vi "Preprocessing.vi"() -> (0 "Timestamp":dbl[](array[numeric]), 1 "Potência instantänea A":dbl[](array[numeric]), 2 "Potência Ativa B":dbl[](graph), 3 "Potência Ativa C":dbl[](graph))   [LabVIEW 2020]
uses:
  <vilib>/numeric/Random Number (Range) U64.vi
  <vilib>/numeric/Random Number (Range) DBL.vi
  <vilib>/numeric/sub_Random U32.vi
panel:
  out "Fator de potência":dbl
  in  "Limite inferior FP":dbl
  in  "Limite superior FP":dbl=100.0
  out "Corrente A":dynamicdata(graph)
  out "Tensão  C":dynamicdata(graph)
  out "Corrente C":dynamicdata(graph)
  out "Tensão B":dynamicdata(graph)
  out "Corrente B":dynamicdata(graph)
  out "Potência Ativa A":dbl[](graph)
  out "Corrente A":dbl[](array[numeric])
  out "Tensão A":dynamicdata(graph)
  out "Tensão A":dbl[](array[numeric])
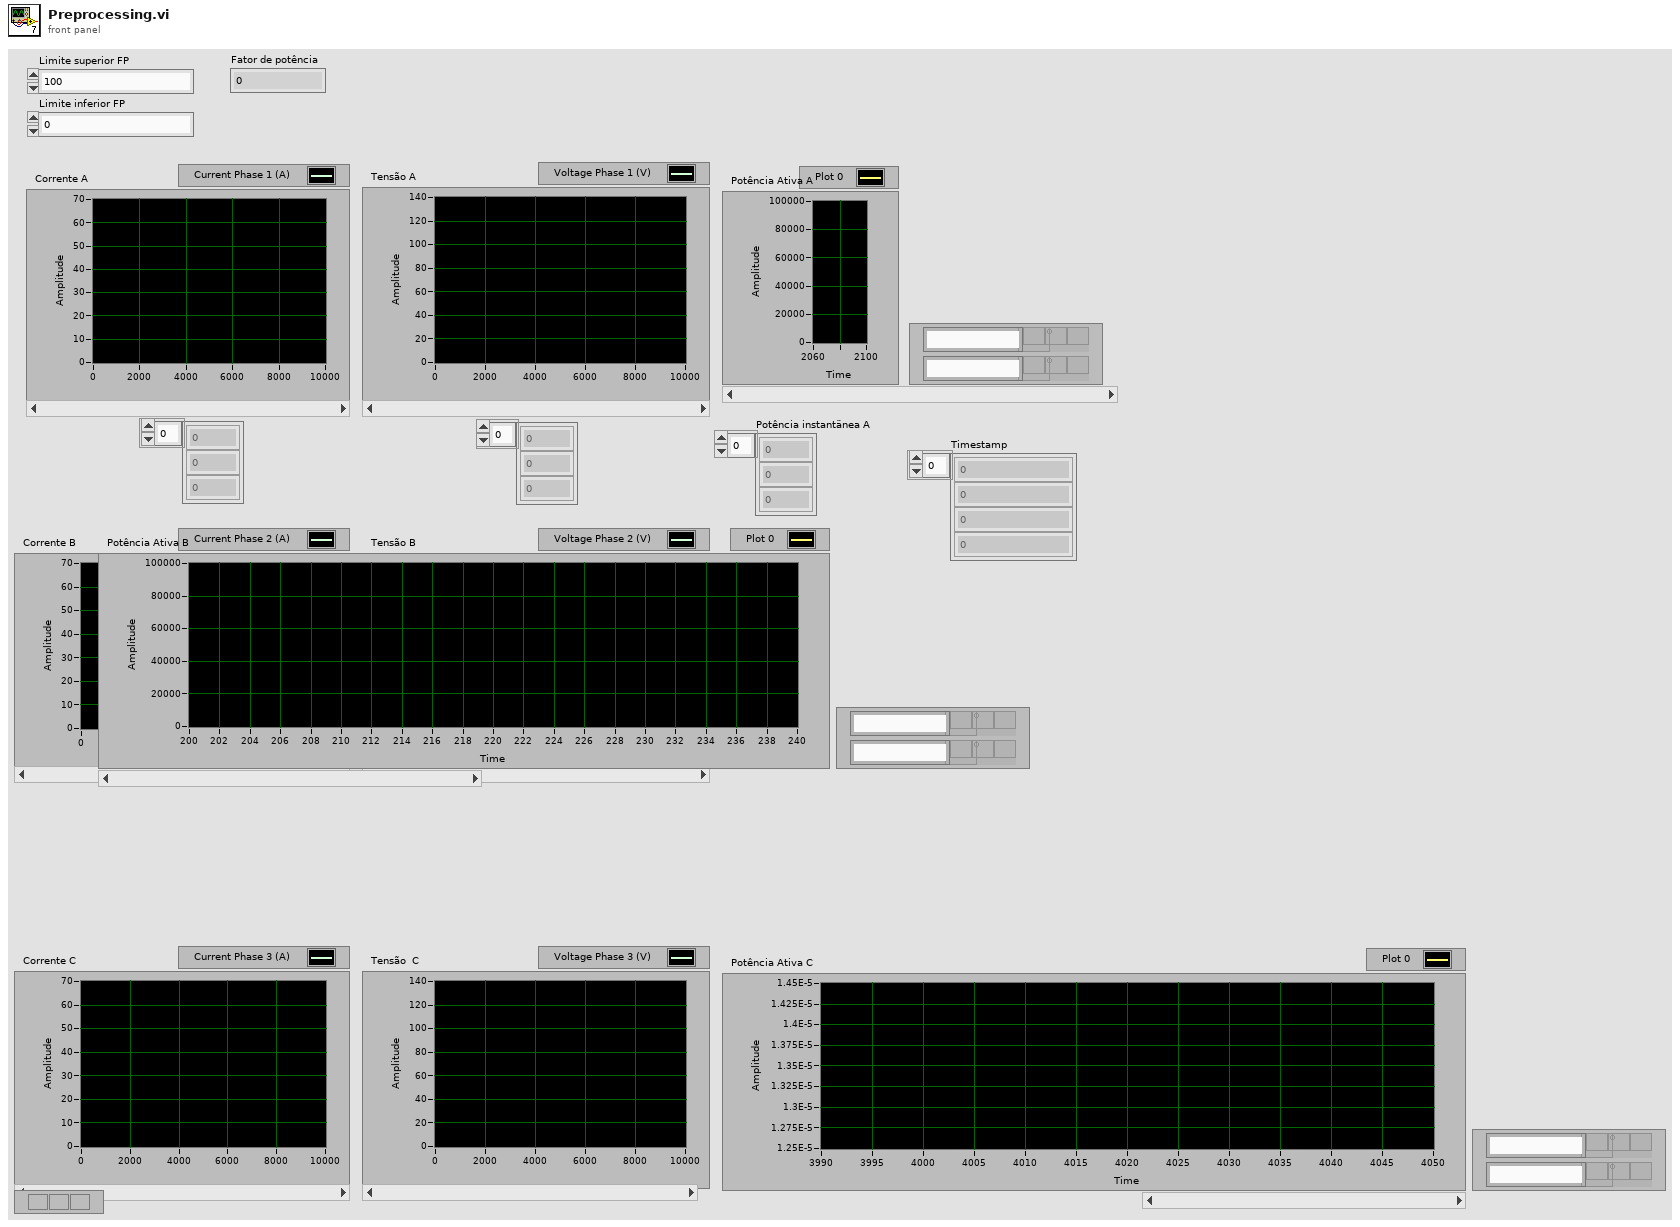
[diagram p1: front panel]
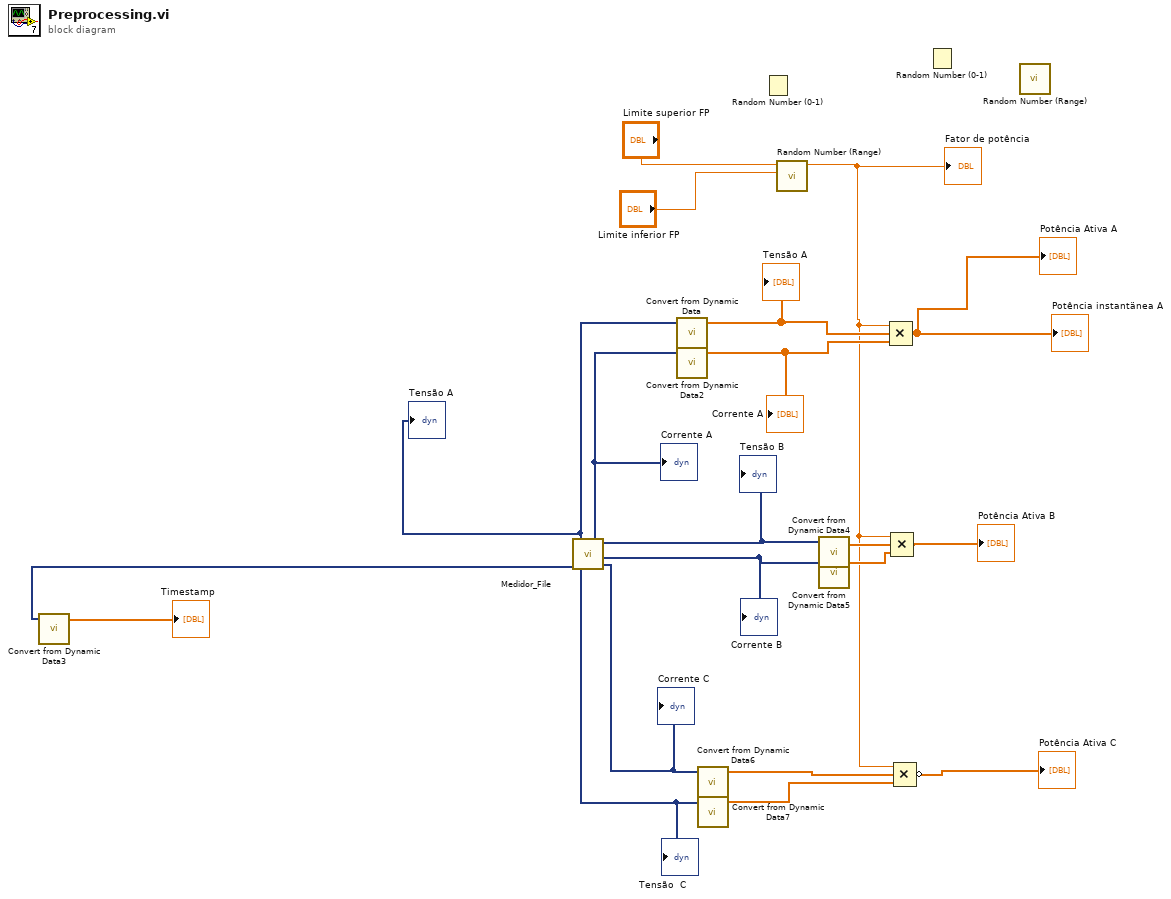
[diagram p0: block diagram]
diagram:
  n1 = call "Medidor_File.vi"() -> ("Corrente Fase C"=w9:dynamicdata, "Corrente Fase B"=w15:dynamicdata, "Corrente Fase A"=w4:dynamicdata, "TimeStamp"=w17:dynamicdata, "Tensão Fase C"=w10:dynamicdata, "Tensão Fase B"=w14:dynamicdata, "Tensão Fase A"=w20:dynamicdata)
  "Tensão A" <- w20
  "Corrente B" <- w15
  "Tensão B" <- w14
  "Corrente C" <- w9
  "Tensão  C" <- w10
  "Corrente A" <- w4
  n2 = call "Convert from Dynamic Data3"("Dynamic Data Type"=w17) -> ("Array"=→"Timestamp":dbl[])  [unwired: 3 in]
  n3 = call "Convert from Dynamic Data"("Dynamic Data Type"=w20) -> ("Array"=w19:dbl[])  [unwired: 3 in]
  "Tensão A" <- w19
  n4 = call "Convert from Dynamic Data2"("Dynamic Data Type"=w4) -> ("Array"=w18:dbl[])  [unwired: 3 in]
  "Corrente A" <- w18
  n5 = call "Convert from Dynamic Data6"("Dynamic Data Type"=w9) -> ("Array"=w8:dbl[])  [unwired: 3 in]
  n6 = call "Convert from Dynamic Data7"("Dynamic Data Type"=w10) -> ("Array"=w7:dbl[])  [unwired: 3 in]
  n7 = Random Number (0-1)() -> ()  [unwired: 1 out]
  n8 = call-poly <vilib>:"Random Number (Range).vi"("lower bound (0)"="Limite inferior FP", "upper bound (100)"="Limite superior FP") -> ("number"=w1:dbl)  [unwired: 9 in]
  "Fator de potência" <- w1
  n9 = call "Convert from Dynamic Data4"("Dynamic Data Type"=w14) -> ("Array"=w13:dbl[])  [unwired: 3 in]
  n10 = call "Convert from Dynamic Data5"("Dynamic Data Type"=w15) -> ("Array"=w12:dbl[])  [unwired: 3 in]
  n11 = Compound Arithmetic op=MULTIPLY(w1, w19, w18) -> (→"Potência instantänea A" →"Potência Ativa A":dbl[])
  n12 = Compound Arithmetic op=MULTIPLY(w1, w13, w12) -> (→"Potência Ativa B":dbl[])
  n13 = Compound Arithmetic op=MULTIPLY(w1, w8, w7) -> (invert →"Potência Ativa C":dbl[])
  n14 = Random Number (0-1)() -> ()  [unwired: 1 out]
  n15 = call-poly <vilib>:"Random Number (Range).vi"() -> ()  [unwired: 11 in, 1 out]
